vi "SampInterval.vi"(3 "Sampling Rate":u16(ring)) -> (0 "Sampling Rate (MHz)":dbl, 1 "time (s)":dbl format="%.2e")   [LabVIEW 2022 SP3]
uses:
  Motion Controllers/-MotionRoutines/MotionGlobals.vi
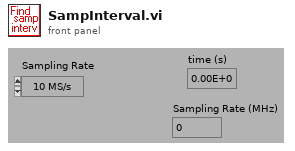
[diagram p1: front panel]
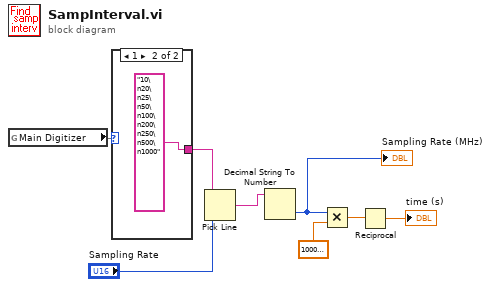
[diagram p0: block diagram]
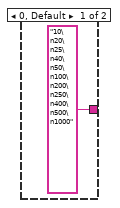
[diagram p2: hidden frame]
diagram:
  n1 = global read "MotionGlobals.vi" "Main Digitizer"() -> (w1)
  n2 = case shown="1" w1 {
    tunnel: ["10\n20\n25\n40\n50\n100\n200\n250\n400\n500\n1000" "10\n20\n25\n50\n100\n200\n250\n500\n1000"] -> w8
    frame 0, Default {
    }
    frame 1 {
    }
  }
  n3 = Pick Line(multi-line string=w8, line index="Sampling Rate") -> (output string=w7:string)  [unwired: 1 out]
  n4 = Decimal String To Number(string=w7) -> (number=w6:i32)  [unwired: 3 out]
  "Sampling Rate (MHz)" <- w6
  n5 = Multiply(x=w6, y=1000000.0) -> (x*y=w4:dbl)
  n6 = Reciprocal(x=w4) -> (1/x=→"time (s)":dbl)
